vi "Station.vi"() -> ()   [LabVIEW 2016]
uses:
  Station.Data.ctl
  Station.State.ctl
  Sequence/Sequence.State.ctl
  Sequence/Sequence.Test.BreakReason.ctl
  Sequence/Sequence.Test.BreakSource.ctl
  Drivers/FestoCPX/Station/FestoCPX.Station.ProdPresent.ctl
  Drivers/FestoCPX/Station/FestoCPX.Station.EmgState.ctl
  Sequence/Sequence.UserData.ctl
  Sequence/Sequence.MainMode.ctl
  Gui/MainGui.TestOptions.ctl
  Station.Home.Status.Bits.ctl
  Station.Action.ctl
  Drivers/FestoCPX/Station/FestoCPX.Station.TowerLed.Color.ctl
  tools/CitTemplate/citTemplate.errData.ctl
  tools/EventLog/EventLog.EventSource.ctl
  Drivers/FestoCPX/FestoCPX.DO.Signal.ctl
  tools/Translator/Translator.Message.ctl
  Logger/Logger.Variant.Sets.ctl
  Station.Changeover.State.vi
  Station.Plate.Properties.ctl
  Sequence/Sequence.Code.SerialFormat.ctl
  Drivers/V7310/LowLevel/V7310.Job.Sets.ctl
  Drivers/FestoCPX/Station/FestoCPX.Station.ButtonsState.ctl
  Drivers/FestoCPX/Station/FestoCPX.Station.ButtonLed.ctl
  Sequence/Sequence.UserAction.ctl
  Sequence/Sequence.Step.Status.ctl
  Drivers/FestoCPX/Station/FestoCPX.Station.TowerHorn.Fglb.Action.ctl
  Global/ApplicationGlobal.vi
  Station.Global.vi
  tools/Config/Config.Global.vi
  Sequence/Sequence.Global.vi
panel:
  out "action":T1=enum."--- Station ---"
  out "Data":T2
  out "_loop":i32(ring)=4
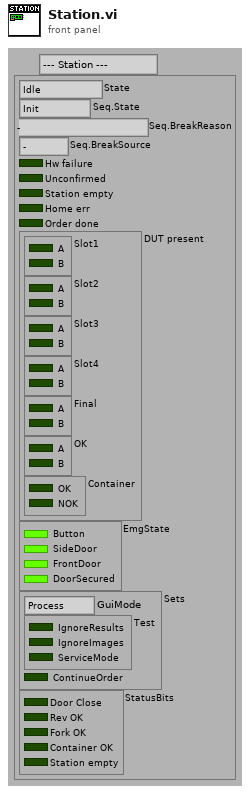
[diagram p1: front panel]
types:
  T1 = typedef "Station.Action.ctl" = enum32{"idle", "constructor", "destructor", "--- Station ---", "Hardware.Init", "Status.Update", "Status.Clear", "Order", "Init", "Ready", "Start", "Run", "Stop", "Error", "Home", "Done", "Seq.Run", "Seq.Done", "Tower.Update", "Mode.Select", "Emg", "Emg.Reset", "Emg.Check", "Home.Check", "Prod.Check", "Butt.Check"}
  T2 = typedef "Station.Data.ctl" = cluster{"State":T3, "Seq.State":T4, "Seq.BreakReason":T5, "Seq.BreakSource":T6, "Hw failure":bool, "Unconfirmed":bool, "Station empty":bool, "Home err":bool, "Order done":bool, "DUT present":T7, "EmgState":T8, "Sets":T9, "StatusBits":T12}
  T3 = typedef "Station.State.ctl" = enum16{"Idle", "Ready", "Run", "Stop", "Error", "Home", "Done", "Emg"}
  T4 = typedef "Sequence.State.ctl" = enum16{"Init", "Idle", "Home", "Work", "Run", "Pause"}
  T5 = typedef "Sequence.Test.BreakReason.ctl" = enum16{"-", "NOK container", "OK container", "Rev empty", "Rev missing", "Rev wrong", "Fork missing", "Fork wrong", "NOK limit", "Unload failure", "Single slot", "Part done", "Err: Prod move work", "Err: Prod move home", "Err: Prod lift work", "Err: Prod lift home", "Err: Prod Arm Work", "Err: Prod Arm NOK", "Err: Prod Arm OK", "Err: Prod NOK suck", "Err: Prod NOK drop", "Err: Prod OK missing", "Err: Prod OK suck", "Err: Prod OK drop"}
  T6 = typedef "Sequence.Test.BreakSource.ctl" = enum16{"-", "A", "B", "A/B"}
  T7 = typedef "FestoCPX.Station.ProdPresent.ctl" = cluster{"Slot1":cluster{"A":bool, "B":bool}, "Slot2":cluster{"A":bool, "B":bool}, "Slot3":cluster{"A":bool, "B":bool}, "Slot4":cluster{"A":bool, "B":bool}, "Final":cluster{"A":bool, "B":bool}, "OK":cluster{"A":bool, "B":bool}, "Container":cluster{"OK":bool, "NOK":bool}}
  T8 = typedef "FestoCPX.Station.EmgState.ctl" = cluster{"Button":bool, "SideDoor":bool, "FrontDoor":bool, "DoorSecured":bool}
  T9 = typedef "Sequence.UserData.ctl" = cluster{"GuiMode":T10, "Test":T11, "ContinueOrder":bool}
  T10 = typedef "Sequence.MainMode.ctl" = enum16{"Process", "Base", "Order", "Manual", "Logs", "Results", "Stats", "DMC Config"}
  T11 = typedef "MainGui.TestOptions.ctl" = cluster{"IgnoreResults":bool, "IgnoreImages":bool, "ServiceMode":bool}
  T12 = typedef "Station.Home.Status.Bits.ctl" = cluster{"Door Close":bool, "Rev OK":bool, "Fork OK":bool, "Container OK":bool, "Station empty":bool}
  T13 = typedef "FestoCPX.Station.TowerLed.Color.ctl" = enum16{"off", "red", "orange", "green", "green/orange"}
  T14 = typedef "citTemplate.errData.ctl" = cluster{"ts":timestamp, "src":T15, "instance":i32, "action":string, "error":errorcluster, "unconfirmed":bool}
  T15 = typedef "EventLog.EventSource.ctl" = enum16{"All", "Gui", "Ref", "File", "Arch", "Seq", "CPX", "DB", "Laser", "Scan.P", "Scan.O"}
  T16 = typedef "FestoCPX.DO.Signal.ctl" = enum16{"Safety Reset", "Air Main Valve", "Door Lock", "Button LED Start", "Button LED Stop", "Button LED Control", "Traffic LED Red", "Traffic LED Orange", "Traffic LED Green", "Horn", "Laser Interlock", "Laser Trigger", "Laser Fume Extractor", "Product Suction Gripper Slot 1 A", "Product Suction Gripper Slot 1 B", "Product Suction Gripper Slot 2 A", "Product Suction Gripper Slot 2 B", "Product Suction Gripper Slot 3 A", "Product Suction Gripper Slot 3 B", "Product Suction Gripper Slot 4 A", "Product Suction Gripper Slot 4 B", "Product Suction Gripper Final A", "Product Suction Gripper Final B", "Lamp", "Q1 Product Move Work", "Q1 Product Move Home", "Q2 Table Turn Work", "Q2 Table Turn Home", "Q3 Product Lift A", "Q3 Product Lift B", "Q4 Product Arm OK", "Q4 Product Arm NOK", "Q5 Product Arm Work", "Q6 Product BlowOut A", "Q6 Product BlowOut B"}
  T17 = typedef "Translator.Message.ctl" = enum16{"-", "Event confirmed", "Log out", "Log in", "Shutdown", "Cancel", "Start", "Begin time", "End time", "Duration", "Service Mode", "Ignore Results", "Serial Format", "On", "Off", "OK", "NOK", "NOK %s", "Home", "Work", "Close", "Open", "In progress...", "Missing", "Empty", "Hardware failure", "Initial", "Default", "Total", "Out of range", "Free disk space is below 1GB - contact technician", "Error %d >> %s", "Error %d >> %s >> %s", "Msg %d >> %s", "Laser msg %d %s", "Laser cmd error %s %d", "Laser cmd failed %s", "Laser cmd warning %s", "Laser disconnected", "Laser status %s", "Laser already started", "Laser job unkonwn %s", "Laser job missing %s", "Laser job select failure %s", "Unable to start laser printing (%s)", "Unable to stop laser printing (%s)", "Laser marking aborted", "Laser marking timeout", "Unable to reset Laser Interlock (%s)", "Unable to trigger Laser. Laser not ready (%s)", "Laser job '%s' coordinates not configured", "Starting %s", "Quitting %s", "Configured", "Initializing", "Quitting", "Loading", "Loaded %d results", "Loaded %d events", "Running", "Stopped", "Summary", "Laser", "Do you want to continue?", "Do you want to delete the configuration?", "The configuration is being used by an order. Unable to delete!", "Press confirm button", "Station is not based. Do you want to exit?", "Station requires changeover. Do you want to run the test?", "Test options are not set as default. Do you want to continue?", "Formatting of WabcoNo is disabled. Do you want to continue?", "Product not detected. Do you want to continue?", "Product scan failed. Do you want to continue?", "Calibration", "Log out?", "System", "All", "IDLE", "Translating...%s", "Not found", "Alarm %s", "Run", "Skip", "Abort", "Repeat", "Please wait...", "Database disconnected", "Database disconnected - changeover disabled!", "Login to database successful", "Login to database failed: %d; %s", "Unable to check the product status of reference %d - database disconnected", "Unable to set the product status of reference %d - database disconnected", "Variant file backup %s", "Read variant (%s)", "Result", "Station armed!", "Station requires changeover!", "Select reference number...", "EMERGENCY BUTTON - press Control button", "EMERGENCY DOOR - press Control button", "Resetting Emergency...", "Unable to reset safety circuit - Emergency Button pressed", "Unable to reset safety circuit - Emergency Side Door open", "Station not based", "Station based", "Station not empty", "Station basing...", "No order", "Press Start to begin new order", "Scanning new order", "Order NOK. Correct or scan again", "Order OK. Press Accept", "Order ready", "Revolver incorrect", "Fork incorrect", "Revolver missing", "Revolver empty", "Container missing", "Offline results", "Offline statistics", "Updating statistics %.1f %%", "DMC Configurator", "Door open", "Close the front door", "Press start button", "Done. Open the front door", "Running...", "Running...%.1f %%", "Pause %s", "Pause %s. NOK container missing", "Pause %s. OK container missing", "Pause %s. Revolver empty", "Pause %s. Revolver missing", "Pause %s. Revolver incorrect", "Pause %s. Fork missing", "Pause %s. Fork incorrect", "Pause %s. Too many failures", "Pause %s. Unloading failure", "Pause %s. One slot is not working", "Pause %s. Part order is done. Empty OK container", "Pause %s. Unable to move product to slot", "Pause %s. Unable to move back product pusher", "Pause %s. Unable to lift product", "Pause %s. Unable to move back product lifter", "Pause %s. Unable to move product arm to Work", "Pause %s. Unable to move product arm to NOK", "Pause %s. Unable to move product arm to OK", "Pause %s. Unable to unsuck the NOK product", "Pause %s. Unable to drop the NOK product", "Pause %s. Product OK missing", "Pause %s. Unable to unsuck the OK product", "Pause %s. Unable to drop the OK product", "Stopping...", "File '%s' is missing", "File '%s' is broken", "File '%s' is running", "Log file started (%s)", "Log file ended (%s)", "Log file stopped (%s)", "Log file ignored (%s)", "Log file exported (%s)", "Log file export failed (%s)", "Wrong serial number in log file", "Wrong reference number in log file", "Test steps are missing", "%s = %.3f", "Process param '%s' not found in DB", "Process param '%s' wrong order", "Process param '%s' value %.3f out of limits (%.3f; %.3f)", "Step%d param '%s' not found in DB", "Step%d param '%s' wrong order", "Step%d param '%s' value %.3f out of limits (%.3f; %.3f)", "Step%d EV '%s' not found in DB", "Step%d EV '%s' wrong order", "\"%s\" not found in DB", "\"%s\" wrong order", "\"%s\" value %.3f out of limits (%.3f; %.3f)", "\"%s\" not found in software", "Process init (%s)", "Process started", "Process restarted", "Process run", "Process done", "Process done - remove OK container", "Process aborted", "Process aborted at work", "Process aborted at home", "Process error", "Process error at home", "Process error at work", "Process close", "Process pause", "Process continue", "Process door open", "Process door close", "Process pause at slot %s due to %s", "Select plate from the order to process", "Do you want to start the process?", "Do you want to continue the process?", "There is unfinished order. Do you want to put the new order?", "Product %s %d OK", "Product %s %d NOK", "Unable to unload the slot %s. Product missing in the slot", "Unable to unload the slot %s. Product already in the arm", "Unable to accept the product as OK. Product missing in slot %s", "Unable to accept the product as OK. Product could not drop into the container at slot %s", "Unable to accept the product as NOK. Product could not drop into the container at slot %s", "Scan failed. Error %s", "Scan failed. Scanner disconnected", "Scan failed. Wrong Wabco number %d, limit (%d,%d)", "Scan failed. Wrong serial number %d, limit (%d,%d)", "Scan failed. Wrong date %d, limit (%d,%d)", "Scan failed. Wrong product wabco number %d (expected %d)", "Scan failed. Wrong product serial number %d (expected > 0)", "Scan OK %s", "Scan failed. Unable to determine table position (%s)", "Scan failed. Timeout", "Tune failed. Scanner disconnected", "Tune failed. Timeout", "%s = %d", "%s = %d->%d", "Unable to set %s = %.2f - Air Pressure Inside off", "Unable to set digital output '%s' = %d", "Unable to activate air pressure inside - timeout", "Unable to activate air pressure inside - aborted", "Unable to switch on Air Main Valve - Air Pressure Inlet off", "Unable to switch on Air Main Valve - Door open", "Unable to switch off Air Main Valve - timeout", "Unable to switch off Air Main Valve - aborted", "Unable to rotate Table - timeout", "Unable to rotate Table - aborted", "Unable to rotate Table - Product Move not in Home position", "Unable to rotate Table - Air Pressure Inside off", "Unable to rotate Table - Product Lift A not in Home position", "Unable to rotate Table - Product Lift B not in Home position", "Unable to rotate Table - unlock before movement timeout", "Unable to rotate Table - lock after movement timeout", "Unable to move Table Lock to %s position - timeout", "Unable to move Table Lock to %s position - aborted", "Unable to move Table Lock to %s position - Air Pressure Inside off", "Unable to move Table Lock to %s position - Table not in position", "Unable to move Product Lift A to %s position - timeout", "Unable to move Product Lift B to %s position - timeout", "Unable to move Product Lift A to %s position - aborted", "Unable to move Product Lift B to %s position - aborted", "Unable to move Product Lift A to %s position - Air Pressure Inside off", "Unable to move Product Lift B to %s position - Air Pressure Inside off", "Unable to move Product Lift A to %s position - Table not locked", "Unable to move Product Lift B to %s position - Table not locked", "Unable to move Product Lift A to %s position - Product Arm not in Work position", "Unable to move Product Lift B to %s position - Product Arm not in Work position", "Unable to set Product Suction Gripper %s to %s - timeout", "Unable to set Product Suction Gripper %s to %s - aborted", "Unable to set Product Suction Gripper %s to %s - Air Pressure Inside off", "Unable to set Product Suction Gripper %s to %s - Table slot unkown", "Unable to move Product Arm to %s position - timeout", "Unable to move Product Arm to %s position - aborted", "Unable to move Product Arm to %s position - Air Pressure Inside off", "Unable to move Product Arm to %s position - Product Lift A not in Home position", "Unable to move Product Arm to %s position - Product Lift B not in Home position", "Unable to move Product to %s position - timeout", "Unable to move Product to %s position - aborted", "Unable to move Product to %s position - Air Pressure Inside off", "Unable to move Product to %s position - Table not in position"}
  T18 = typedef "Logger.Variant.Sets.ctl" = cluster{"State":T19, "ImgPath":path, "WabcoPlate":string, "WabcoProduct":string, "ClientProduct":string, "ClientPlate":string, "TotalQuantity":u16, "OrderQuantity":u16, "Serial":i32, "Wabco":T20, "Client":T20}
  T19 = typedef "Station.Changeover.State.vi" = enum16{"Init", "Scaning", "NOK", "Wait for ack", "Ready"}
  T20 = typedef "Station.Plate.Properties.ctl" = cluster{"LaserJob":string, "AdditionalTxt":string, "FactoryCode":string, "RevID":u8, "ForkID":u8, "FailuresLimit":u16, "GlobalCnt":i32, "Bank":u8, "SerialFormat":T21, "CoordA":T22, "CoordB":T22, "DMCconfig":i32}
  T21 = typedef "Sequence.Code.SerialFormat.ctl" = enum8{"", "6 dig", "7 dig"}
  T22 = typedef "V7310.Job.Sets.ctl" = cluster{"X":dbl, "Y":dbl, "Angle":dbl}
  T23 = typedef "FestoCPX.Station.ButtonsState.ctl" = cluster{"Start":bool, "Stop":bool, "Control":bool}
  T24 = typedef "Sequence.UserAction.ctl" = enum16{"-", "Stop", "Pause", "Continue", "Next"}
  T25 = typedef "FestoCPX.Station.ButtonLed.ctl" = enum16{"Start", "Stop", "Control"}
  T26 = cluster{"State":T4, "PauseReason":T5, "BreakSource":T6}
  T27 = typedef "Sequence.Step.Status.ctl" = enum16{"-", "Pending", "Running", "Skipped", "Passed", "Failed", "Done", "Error", "Aborted", "Stopped"}
  T28 = cluster{"State":T4, "Status":T27, "order done":bool}
  T29 = typedef "FestoCPX.Station.TowerHorn.Fglb.Action.ctl" = enum16{"init", "set", "get"}
  T30 = typedef "citTemplate.notifierHandle.ctl" = refnum<notifier>
  T31 = cluster{"Arguments":variant[], "msg":T17, "BgColor":u32, u32, "Blink":bool}
  T32 = typedef "Sequence.Data.ctl" = cluster{"BeginTS":timestamp, "EndTS":timestamp, "State":T4, "Status.Work":T27, "Status.Process":T27, "Status.Home":T27, "Status.Wabco":T27, "Status.Client":T27, "BreakReason":T5, "BreakSource":T6, "DoorLock":bool, "Status.Prod":T33[], "UserAction":T37, "UserData":T9, "Error":errorcluster, "Code":T38, "Rotations":i32, "ProdIdx":i32, "ProdDone":T33[], "PrintedSerials-Wabco":i32[], "PrintedSerials-Client":i32[], "Counters-Wabco":T40, "Counters-Client":T40}
  T33 = typedef "Sequence.Test.Status.ctl" = cluster{"Slot":T34, "A":T36, "B":T36}
  T34 = typedef "Sequence.Slot.StatusData.ctl" = cluster{"ID":i32, "Unload":T35, "TS":timestamp, "duration":u32}
  T35 = typedef "Sequence.Test.Unload.Status.ctl" = enum16{"init", "check NOK", "check OK", "wait on NOK", "wait on OK", "wait on Unload", "done"}
  T36 = typedef "Sequence.Prod.StatusData.ctl" = cluster{"status":T27, "pause":T5, "present":bool, "printed":bool, "scanned":bool, "tuned":bool, "removed":bool, "LaserVariables":string[], "ScanerReadOut":string, "path":path, "corners":cluster{"X":i32, "Y":i32}[], "verification":u8}
  T37 = typedef "Sequence.UserActions.ctl" = cluster{"Stop":bool, "Pause":bool, "Next":bool}
  T38 = typedef "Sequence.Code.Sets.ctl" = cluster{"Ready":bool, "DoubleOrder":bool, "OrderDone":bool, "AllowSingleSlot":bool, "CheckDM":bool, "ThresholdA":u8, "ThresholdB":u8, "Plate":T39, "ImgPath":path, "Variant":T18}
  T39 = typedef "Sequence.PlateType.ctl" = enum16{"Wabco", "Client"}
  T40 = typedef "Sequence.Counters.ctl" = cluster{"Expected":u16, "Done":u16, "OK":u16, "NOK":u16, "NOKlimit":u16, "Part":u16, "PartOK":u16}
  T41 = typedef "Station.Buttons.ctl" = cluster{"Start":bool, "Stop":bool, "Control":bool}
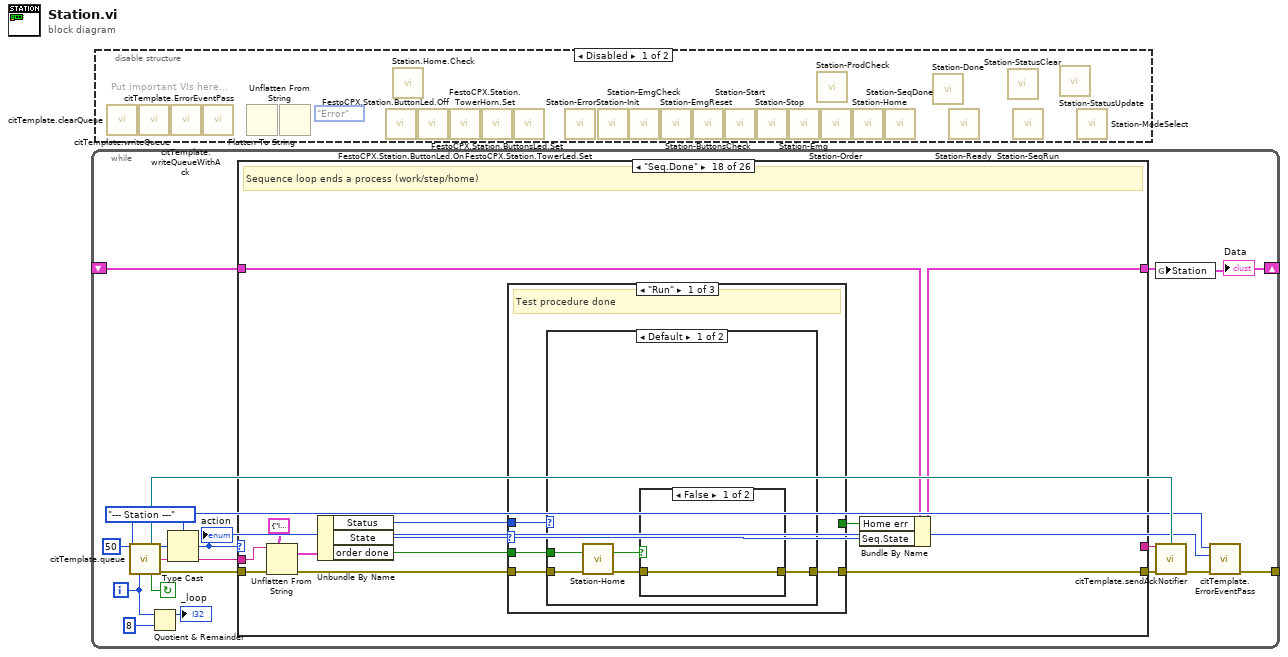
[diagram p0: block diagram]
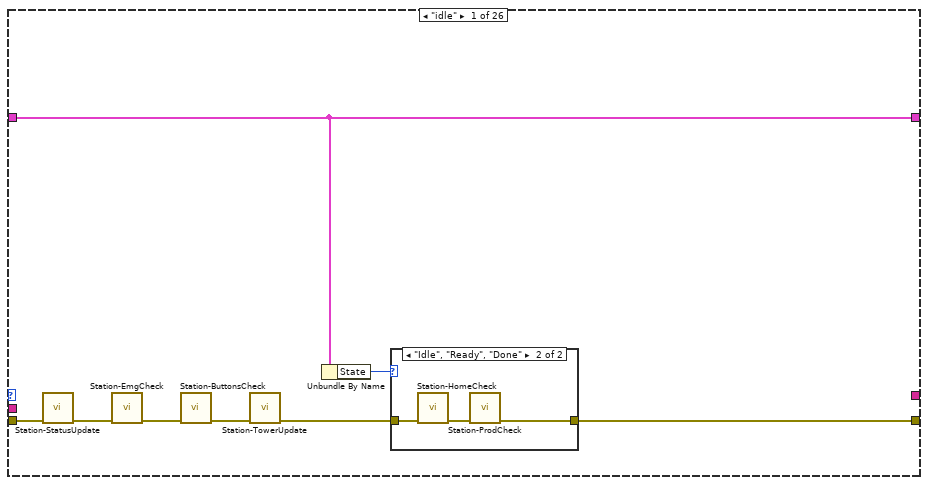
[diagram p3: hidden frame]
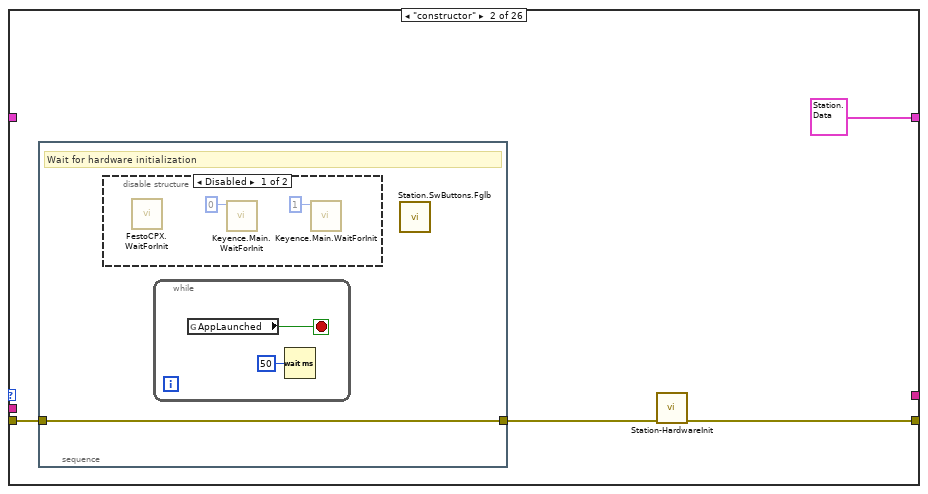
[diagram p5: hidden frame]
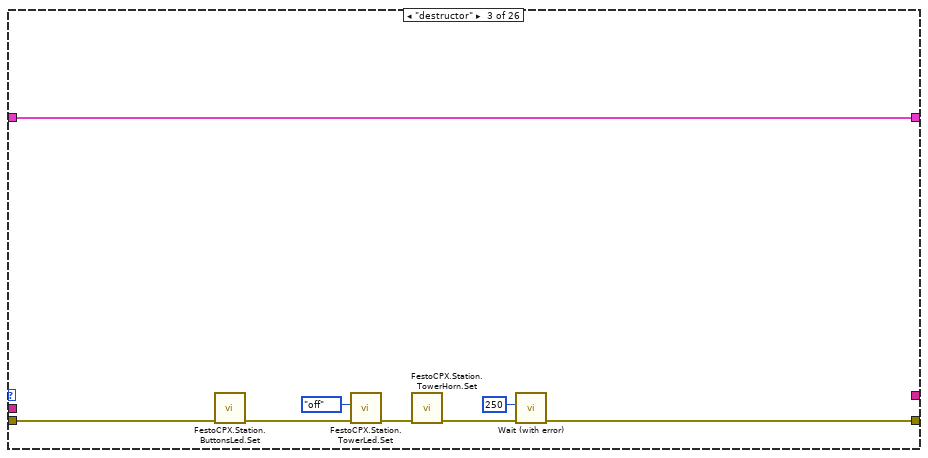
[diagram p7: hidden frame]
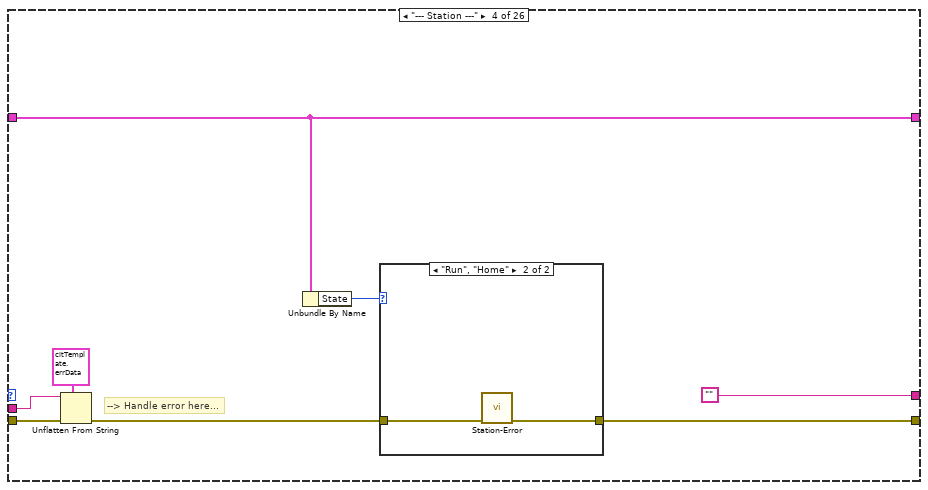
[diagram p8: hidden frame]
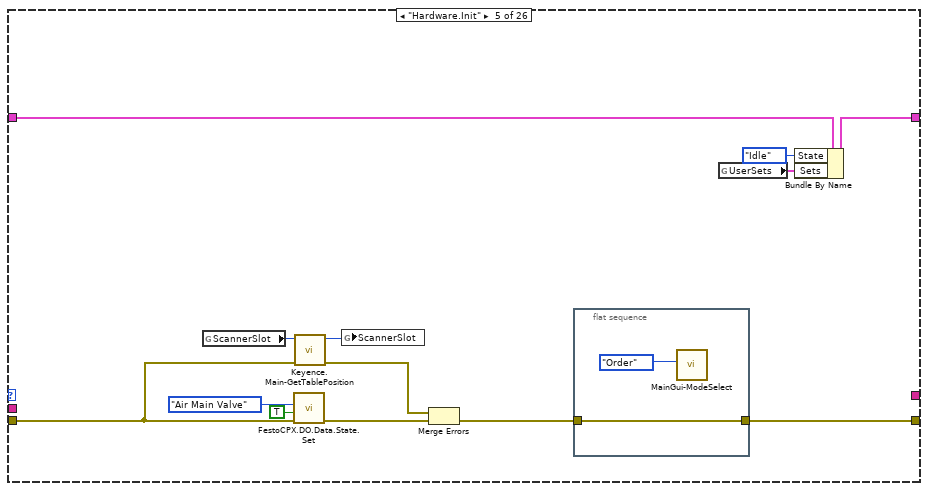
[diagram p10: hidden frame]
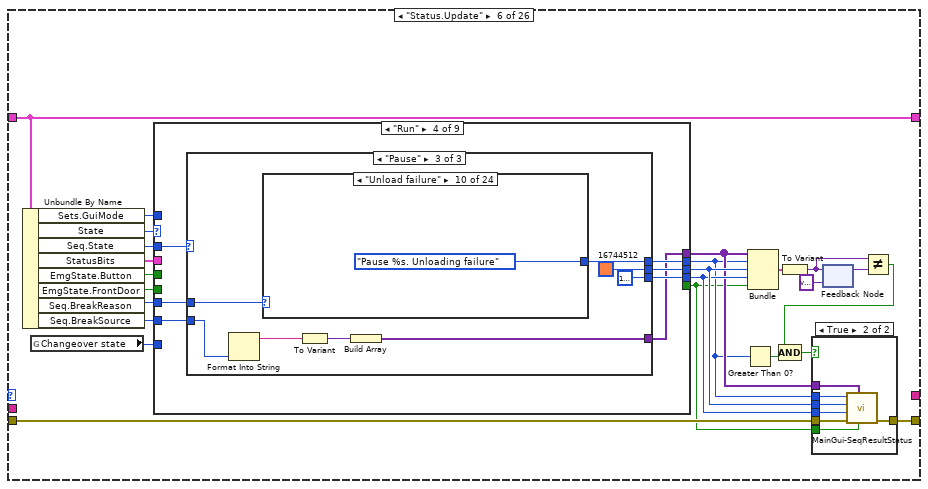
[diagram p11: hidden frame]
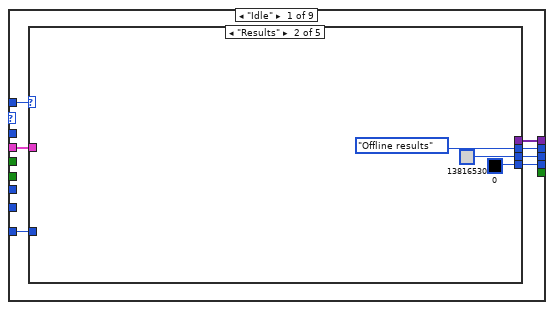
[diagram p13: hidden frame]
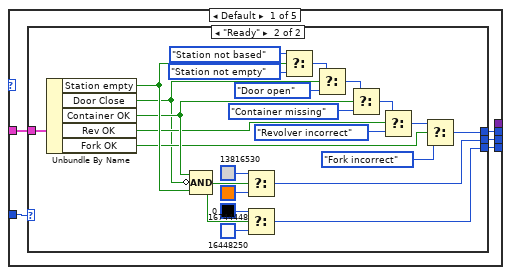
[diagram p14: hidden frame]
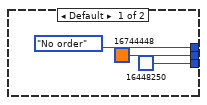
[diagram p15: hidden frame]
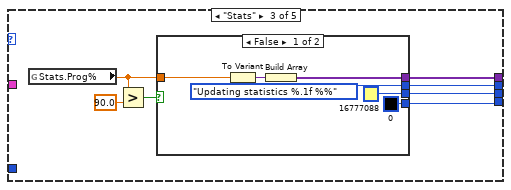
[diagram p16: hidden frame]
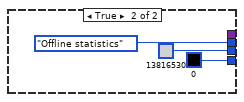
[diagram p17: hidden frame]
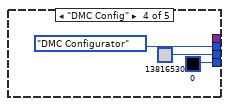
[diagram p18: hidden frame]
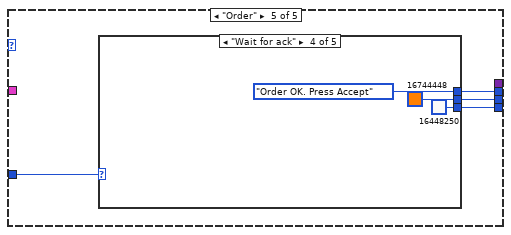
[diagram p19: hidden frame]
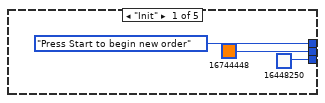
[diagram p20: hidden frame]
diagram:
  n1 = while {
    tunnel: [w5] -> _
    shift-right: [w2] -> _
    shift-left: _ -> [w3]
    i -> [w7]
    stop <- w13 continue-if-true
    w10 = Station.Action."--- Station ---" ("Action")
    n2 = call "citTemplate.queue.vi"("ms timeout (250 ms)"=50, "event enum"=w10, "iteration (-1)"=w7) -> ("notifierHandle out"=w12:T30, "event out"=w16:u32, "(flatten) data out"=w15:string, "continue"=w13:bool, "error out"=w14:errorcluster)  [unwired: 2 in, 6 out]
    n3 = Quotient & Remainder(x=w7, y=8) -> (x-y*floor(x/y)=→"_loop":i32)  [unwired: 1 out]
    n4 = Type Cast(type=w10, x=w16) -> (*(type *) &x=w6:T1)
    "action" <- w6
    n5 = case shown="\"Seq.Done\"" w6 {
      tunnel: w15 -> [_ _ _ w52 _ _ _ w304 _ _ _ _ _ _ _ _ w443 w466 _ w525 _ _ _ _ _ _]
      tunnel: w14 -> [w24 w32 w38 w51 w65 w89 w289 w311 w335 w345 w365 w388 w399 w405 w417 w430 w444 w467 w502 w526 w549 w568 w587 w613 w643 w663]
      tunnel: [_ _ _ "" _ _ _ _ _ _ _ _ _ _ _ _ _ _ _ _ _ _ _ _ _ _] -> w11
      tunnel: [w22 T2 {"State"=enum."Idle", "Seq.State"=enum."Init", "Seq.BreakReason"=enum."-", "Seq.BreakSource"=enum."-", "Hw failure"=FALSE, "Unconfirmed"=FALSE, "Station empty"=FALSE, "Home err"=FALSE, "Order done"=FALSE, "DUT present"={"Slot1"={"A"=FALSE, "B"=FALSE}, "Slot2"={"A"=FALSE, "B"=FALSE}, "Slot3"={"A"=FALSE, "B"=FALSE}, "Slot4"={"A"=FALSE, "B"=FALSE}, "Final"={"A"=FALSE, "B"=FALSE}, "OK"={"A"=FALSE, "B"=FALSE}, "Container"={"OK"=FALSE, "NOK"=FALSE}}, "EmgState"={"Button"=FALSE, "SideDoor"=FALSE, "FrontDoor"=FALSE, "DoorSecured"=FALSE}, "Sets"={"GuiMode"=enum."Process", "Test"={"IgnoreResults"=FALSE, "IgnoreImages"=FALSE, "ServiceMode"=FALSE}, "ContinueOrder"=FALSE}, "StatusBits"={"Door Close"=FALSE, "Rev OK"=FALSE, "Fork OK"=FALSE, "Container OK"=FALSE, "Station empty"=FALSE}} ("Data") w42 w49 w59 w95 w294 w306 w339 w352 w360 w390 w400 w410 w421 w433 w442 w461 w505 w518 w554 w569 w582 w611 w641 w649] -> w2
      tunnel: w3 -> [w22 _ w42 w49 w60 w95 w291 w306 w337 w350 w362 w387 w398 w404 w420 w431 w441 w457 w505 w523 w548 w570 w583 w612 w640 w649]
      tunnel: [w17 w30 w44 w47 w57 w90 w292 w309 w334 w344 w364 w384 w391 w403 w419 w424 w436 w463 w494 w520 w547 w566 w585 w610 w642 w653] -> w1
      frame "idle" {
        n6 = call "Station-StatusUpdate.vi"("error in (no error)"=w24) -> ("error out"=w23:errorcluster)  [unwired: 10 in]
        n7 = call "Station-EmgCheck.vi"("error in (no error)"=w23) -> ("error out"=w20:errorcluster)  [unwired: 10 in]
        n8 = call "Station-ButtonsCheck.vi"("error in (no error)"=w20) -> ("error out"=w19:errorcluster)  [unwired: 10 in]
        n9 = call "Station-TowerUpdate.vi"("error in (no error)"=w19) -> ("error out"=w18:errorcluster)  [unwired: 10 in]
        n10 = Unbundle By Name(w22) -> ("State"=w21:T3)
        n11 = case shown="\"Idle\", \"Ready\", \"Done\"" w21 {
          tunnel: w18 -> [w25 w28]
          tunnel: [w25 w26] -> w17
          frame Default {
          }
          frame "Idle", "Ready", "Done" {
            n12 = call "Station-HomeCheck.vi"("error in (no error)"=w28) -> ("error out"=w27:errorcluster)  [unwired: 10 in]
            n13 = call "Station-ProdCheck.vi"("error in (no error)"=w27) -> ("error out"=w26:errorcluster)  [unwired: 10 in]
          }
        }
      }
      frame "constructor" {
        n14 = stacked-sequence {
          tunnel: w32 -> [w33]
          tunnel: [w33] -> w31
          frame #0 {
            # "Wait for hardware initialization"
            n15 = disable-structure shown="Disabled" {
              frame Disabled {
                n16 = call "FestoCPX.WaitForInit.vi"() -> ()  [unwired: 12 in]
                n17 = call "Keyence.Main.WaitForInit.vi"("idx"=0) -> ()  [unwired: 11 in]
                n18 = call "Keyence.Main.WaitForInit.vi"("idx"=1) -> ()  [unwired: 11 in]
              }
              frame Enabled {
              }
            }
            n19 = while {
              stop <- w35 stop-if-true
              n20 = global read "ApplicationGlobal.vi" "AppLaunched"() -> (w35:bool)
              n21 = Wait (ms)(milliseconds to wait=u32 50) -> ()  [unwired: 1 out]
            }
            n22 = call "Station.SwButtons.Fglb.vi"() -> ()  [unwired: 2 in, 1 out]
          }
        }
        n23 = call "Station-HardwareInit.vi"("error in (no error)"=w31) -> ("error out"=w30:errorcluster)  [unwired: 10 in]
      }
      frame "destructor" {
        n24 = call "FestoCPX.Station.ButtonsLed.Set.vi"("error in"=w38) -> ("error out"=w39:errorcluster)  [unwired: 10 in]
        n25 = call "FestoCPX.Station.TowerLed.Set.vi"("error in"=w39, "Color (off)"=FestoCPX.Station.TowerLed.Color."off") -> ("error out"=w40:errorcluster)  [unwired: 9 in]
        n26 = call "FestoCPX.Station.TowerHorn.Set.vi"("error in"=w40) -> ("error out"=w45:errorcluster)  [unwired: 10 in]
        n27 = call "Wait (with error).vi"("error in (no error)"=w45, "milliseconds to wait"=u32 250) -> ("error out"=w44:errorcluster)  [unwired: 8 in, 1 out]
      }
      frame "--- Station ---" {
        # "--> Handle error here..."
        n28 = Unflatten From String(type=T14 {"ts"=timestamp(0 s since 1904-01-01), "src"=enum."All", "instance"=0, "action"="", "error"={"status"=FALSE, "code"=0, "source"=""}, "unconfirmed"=FALSE} ("ErrData"), binary string=w52, error in (no error)=w51) -> (error out=w46:errorcluster)  [unwired: 4 out]
        n29 = Unbundle By Name(w49) -> ("State"=w48:T3)
        n30 = case shown="\"Run\", \"Home\"" w48 {
          tunnel: w46 -> [w54 w56]
          tunnel: [w54 w55] -> w47
          frame Default {
          }
          frame "Run", "Home" {
            n31 = call "Station-Error.vi"("error in (no error)"=w56) -> ("error out"=w55:errorcluster)  [unwired: 10 in]
          }
        }
      }
      frame "Hardware.Init" {
        n32 = global read "Station.Global.vi" "ScannerSlot"() -> (w67:i32)
        n33 = call "FestoCPX.DO.Data.State.Set.vi"("error in (no error)"=w65, "State"=TRUE, "CPX.DO"=FestoCPX.DO.Signal."Air Main Valve") -> ("error out"=w64:errorcluster)  [unwired: 8 in]
        n34 = call "Keyence.Main-GetTablePosition.vi"("error in (no error)"=w65, "ScannerSlot in"=w67) -> ("error out"=w63:errorcluster, "ScannerSlot out"=w66:i32)  [unwired: 7 in, 1 out]
        n35 = global write "Station.Global.vi" "ScannerSlot"(w66) -> ()
        n36 = Merge Errors(w63, w64) -> (w58:errorcluster)
        n37 = flat-sequence {
          tunnel: w58 -> [w70]
          tunnel: [w70] -> w57
          frame #0 {
            n38 = call "MainGui-ModeSelect.vi"("Mode"=Sequence.MainMode."Order" ("f")) -> ()  [unwired: 10 in, 1 out]
          }
        }
        n39 = global read "Config.Global.vi" "UserSets"() -> (w62:T9)
        n40 = Bundle By Name(cluster=w60, "State"=Station.State."Idle", "Sets"=w62) -> (w59:T2)
      }
      frame "Status.Update" {
        n41 = Unbundle By Name(w95) -> ("Sets.GuiMode"=w76:T10, "State"=w94:T3, "Seq.State"=w77:T4, "StatusBits"=w78:T12, "EmgState.Button"=w81:bool, "EmgState.FrontDoor"=w74:bool, "Seq.BreakReason"=w75:T5, "Seq.BreakSource"=w72:T6)
        n42 = global read "Station.Global.vi" "Changeover state"() -> (w73:T19)
        n43 = case shown="\"Run\"" w94 {
          tunnel: [w110 w189 Translator.Message."Done. Open the front door" ("msg") w235 Translator.Message."Stopping..." ("msg") _ Translator.Message."Station basing..." ("msg") w281 _] -> w85
          tunnel: [w109 w188 u32 16744448 w234 u32 16860 _ u32 16860 u32 16711680 _] -> w88
          tunnel: [w108 w187 u32 16448250 w233 u32 16448250 _ u32 16448250 u32 16777225 _] -> w87
          tunnel: [w104 w184 _ w229 _ _ _ _ variant[] [] ("Arguments")] -> w86
          tunnel: [_ _ _ _ _ _ _ TRUE ("Blink") _] -> w79
          tunnel: w81 -> [_ _ _ _ _ _ _ w282 _]
          tunnel: w78 -> [w107 w186 _ _ _ _ _ _ _]
          tunnel: w77 -> [_ _ _ w232 _ _ _ _ _]
          tunnel: w76 -> [w106 w185 _ _ _ _ _ _ _]
          tunnel: w75 -> [_ _ _ w231 _ _ _ _ _]
          tunnel: w74 -> [_ _ _ _ _ _ _ _ _]
          tunnel: w73 -> [w105 _ _ _ _ _ _ _ _]
          tunnel: w72 -> [_ _ _ w230 _ _ _ _ _]
          frame "Idle" {
            n44 = case shown="\"Results\"" w106 {
              tunnel: [w115 Translator.Message."Offline results" ("msg") w150 Translator.Message."DMC Configurator" ("msg") w168] -> w110
              tunnel: [w114 u32 13816530 w149 u32 13816530 w167] -> w109
              tunnel: [w113 u32 0 w148 u32 0 w166] -> w108
              tunnel: w107 -> [w112 _ _ _ _]
              tunnel: w105 -> [w111 _ _ _ w165]
              tunnel: [_ _ w147 _ _] -> w104
              frame Default {
                n45 = case shown="\"Ready\"" w111 {
                  tunnel: [Translator.Message."No order" ("msg") w120] -> w115
                  tunnel: [u32 16744448 w130] -> w114
                  tunnel: [u32 16448250 w129] -> w113
                  tunnel: w112 -> [_ w128]
                  frame Default {
                  }
                  frame "Ready" {
                    n46 = Unbundle By Name(w128) -> ("Station empty"=w134:bool, "Door Close"=w119:bool, "Container OK"=w127:bool, "Rev OK"=w126:bool, "Fork OK"=w122:bool)
                    n47 = Compound Arithmetic op=AND(w127, invert w119, w134) -> (w131:bool)
                    n48 = Select(t=u32 13816530, s=w131, f=u32 16744448) -> (s? t:f=w130:u32)
                    n49 = Select(t=u32 0, s=w131, f=u32 16448250) -> (s? t:f=w129:u32)
                    n50 = Select(t=Translator.Message."Station not based" ("msg"), s=w134, f=Translator.Message."Station not empty" ("msg")) -> (s? t:f=w139:T17)
                    n51 = Select(t=w139, s=w119, f=Translator.Message."Door open" ("msg")) -> (s? t:f=w140:T17)
                    n52 = Select(t=w140, s=w127, f=Translator.Message."Container missing" ("msg")) -> (s? t:f=w124:T17)
                    n53 = Select(t=w124, s=w126, f=Translator.Message."Revolver incorrect" ("msg")) -> (s? t:f=w123:T17)
                    n54 = Select(t=w123, s=w122, f=Translator.Message."Fork incorrect" ("msg")) -> (s? t:f=w120:T17)
                  }
                }
              }
              frame "Results" {
              }
              frame "Stats" {
                n55 = global read "ApplicationGlobal.vi" "Stats.Prog%"() -> (w146:dbl)
                n56 = Greater?(x=w146, y=90.0) -> (0:w151:bool)
                n57 = case shown="False" w151 {
                  tunnel: [Translator.Message."Updating statistics %.1f %%" ("msg") Translator.Message."Offline statistics" ("msg")] -> w150
                  tunnel: [u32 16777088 u32 13816530] -> w149
                  tunnel: [u32 0 u32 0] -> w148
                  tunnel: [w156 _] -> w147
                  tunnel: w146 -> [w155 _]
                  frame False {
                    n58 = To Variant(anything=w155) -> (Variant=w157:variant)
                    n59 = Build Array(w157) -> (w156:variant[])
                  }
                  frame True {
                  }
                }
              }
              frame "DMC Config" {
              }
              frame "Order" {
                n60 = case shown="\"Wait for ack\"" w165 {
                  tunnel: [Translator.Message."Press Start to begin new order" ("msg") Translator.Message."Order NOK. Correct or scan again" ("msg") Translator.Message."Scanning new order" ("msg") Translator.Message."Order OK. Press Accept" ("msg") Translator.Message."Order ready" ("msg")] -> w168
                  tunnel: [u32 16744448 u32 16744448 u32 16744448 u32 16744448 u32 13816530] -> w167
                  tunnel: [u32 16448250 u32 16448250 u32 16448250 u32 16448250 u32 0] -> w166
                  frame "Init" {
                  }
                  frame "NOK" {
                  }
                  frame "Scaning" {
                  }
                  frame "Wait for ack" {
                  }
                  frame "Ready" {
                  }
                }
              }
            }
          }
          frame "Ready" {
            n61 = case shown="\"Results\"" w185 {
              tunnel: [_ w192 w210 Translator.Message."Station based" ("msg") Translator.Message."Offline results" ("msg") Translator.Message."Press Start to begin new order" ("msg")] -> w189
              tunnel: [_ w190 w209 u32 13816530 u32 13816530 u32 13816530] -> w188
              tunnel: [_ w193 w208 u32 0 u32 0 u32 0] -> w187
              tunnel: w186 -> [_ _ w207 _ _ _]
              tunnel: [_ w191 _ _ _ _] -> w184
              frame Default {
              }
              frame "Stats" {
                n62 = global read "ApplicationGlobal.vi" "Stats.Prog%"() -> (w194:dbl)
                n63 = Greater?(x=w194, y=90.0) -> (0:w195:bool)
                n64 = case shown="False" w195 {
                  tunnel: [Translator.Message."Updating statistics %.1f %%" ("msg") Translator.Message."Offline statistics" ("msg")] -> w192
                  tunnel: [u32 16777088 u32 13816530] -> w190
                  tunnel: [u32 0 u32 0] -> w193
                  tunnel: [w200 _] -> w191
                  tunnel: w194 -> [w199 _]
                  frame False {
                    n65 = To Variant(anything=w199) -> (Variant=w201:variant)
                    n66 = Build Array(w201) -> (w200:variant[])
                  }
                  frame True {
                  }
                }
              }
              frame "Process" {
                n67 = Unbundle By Name(w207) -> ("Door Close"=w206:bool)
                n68 = case shown="False" w206 {
                  tunnel: [Translator.Message."Close the front door" ("msg") Translator.Message."Press start button" ("msg")] -> w210
                  tunnel: [u32 13816530 u32 13816530 ("BgColor")] -> w209
                  tunnel: [u32 0 u32 0] -> w208
                  frame False {
                  }
                  frame True {
                  }
                }
              }
              frame "Base" {
              }
              frame "Results" {
              }
              frame "Order" {
              }
            }
          }
          frame "Done" {
          }
          frame "Run" {
            n69 = case shown="\"Pause\"" w232 {
              tunnel: [Translator.Message."Running..." ("msg") Translator.Message."Running..." ("msg") w247] -> w235
              tunnel: [u32 16860 u32 16860 u32 16744512] -> w234
              tunnel: [u32 16777225 u32 16777225 u32 16777225] -> w233
              tunnel: w231 -> [_ _ w246]
              tunnel: w230 -> [_ _ w245]
              tunnel: [_ _ w242] -> w229
              frame Default {
              }
              frame "Run" {
              }
              frame "Pause" {
                n70 = Format Into String(w245) -> (resulting string=w244:string)  [unwired: 3 in, 1 out]
                n71 = case shown="\"Unload failure\"" w246 {
                  tunnel: [Translator.Message."Pause %s" ("msg") Translator.Message."Pause %s. NOK container missing" ("msg") Translator.Message."Pause %s. OK container missing" ("msg") Translator.Message."Pause %s. Revolver empty" ("msg") Translator.Message."Pause %s. Revolver missing" ("msg") Translator.Message."Pause %s. Revolver incorrect" ("msg") Translator.Message."Pause %s. Fork missing" ("msg") Translator.Message."Pause %s. Fork incorrect" ("msg") Translator.Message."Pause %s. Too many failures" ("msg") Translator.Message."Pause %s. Unloading failure" ("msg") Translator.Message."Pause %s. One slot is not working" ("msg") Translator.Message."Pause %s. Part order is done. Empty OK container" ("msg") Translator.Message."Pause %s. Unable to move product to slot" ("msg") Translator.Message."Pause %s. Unable to move back product pusher" ("msg") Translator.Message."Pause %s. Unable to lift product" ("msg") Translator.Message."Pause %s. Unable to move back product lifter" ("msg") Translator.Message."Pause %s. Unable to move product arm to Work" ("msg") Translator.Message."Pause %s. Unable to move product arm to NOK" ("msg") Translator.Message."Pause %s. Unable to move product arm to OK" ("msg") Translator.Message."Pause %s. Unable to unsuck the NOK product" ("msg") Translator.Message."Pause %s. Unable to drop the NOK product" ("msg") Translator.Message."Pause %s. Product OK missing" ("msg") Translator.Message."Pause %s. Unable to unsuck the OK product" ("msg") Translator.Message."Pause %s. Unable to drop the OK product" ("msg")] -> w247
                  frame "-" {
                  }
                  frame "NOK container" {
                  }
                  frame "OK container" {
                  }
                  frame "Rev empty" {
                  }
                  frame "Rev missing" {
                  }
                  frame "Rev wrong" {
                  }
                  frame "Fork missing" {
                  }
                  frame "Fork wrong" {
                  }
                  frame "NOK limit" {
                  }
                  frame "Unload failure" {
                  }
                  frame "Single slot" {
                  }
                  frame "Part done" {
                  }
                  frame "Err: Prod move work" {
                  }
                  frame "Err: Prod move home" {
                  }
                  frame "Err: Prod lift work" {
                  }
                  frame "Err: Prod lift home" {
                  }
                  frame "Err: Prod Arm Work" {
                  }
                  frame "Err: Prod Arm NOK" {
                  }
                  frame "Err: Prod Arm OK" {
                  }
                  frame "Err: Prod NOK suck" {
                  }
                  frame "Err: Prod NOK drop" {
                  }
                  frame "Err: Prod OK missing" {
                  }
                  frame "Err: Prod OK suck" {
                  }
                  frame "Err: Prod OK drop" {
                  }
                }
                n72 = To Variant(anything=w244) -> (Variant=w243:variant)
                n73 = Build Array(w243) -> (w242:variant[])
              }
            }
          }
          frame "Stop" {
          }
          frame "Error" {
          }
          frame "Home" {
          }
          frame "Emg" {
            n74 = Select(t=Translator.Message."EMERGENCY BUTTON - press Control button" ("msg"), s=w282, f=Translator.Message."EMERGENCY DOOR - press Control button" ("msg")) -> (s? t:f=w281:T17)
          }
          frame Default {
          }
        }
        n75 = Greater Than 0?(x=w85) -> (x > 0?=w84:bool)
        n76 = Bundle("Arguments"=w86, "msg"=w85, "BgColor"=w88, w87, "Blink"=w79) -> (w93:T31)  [unwired: 1 in]
        n77 = To Variant(anything=w93) -> (Variant=w91:variant)
        n78 = feedback-in #1(w91) -> ()
        n79 = feedback #1(variant ("Variant")) -> (w92:variant)
        n80 = Not Equal?(x=w91, y=w92) -> (x != y?=w83:bool)
        n81 = Compound Arithmetic op=AND(w83, w84) -> (w82:bool)
        n82 = case shown="True" w82 {
          tunnel: [w96 w103] -> w90
          tunnel: w89 -> [w96 w102]
          tunnel: w88 -> [_ w101]
          tunnel: w87 -> [_ w100]
          tunnel: w85 -> [_ w99]
          tunnel: w86 -> [_ w98]
          tunnel: w79 -> [_ w97]
          frame False {
          }
          frame True {
            n83 = call "MainGui-SeqResultStatus.vi"("Blink"=w97, "Arguments"=w98, "error in (no error)"=w102, "TxtColor"=w100, "BgColor"=w101, "Msg"=w99) -> ("error out"=w103:errorcluster)  [unwired: 5 in]
          }
        }
      }
      frame "Status.Clear" {
        n84 = call "ErrorHandling.Fglb.Confirm.vi"("error in (no error)"=w289) -> ("error out"=w288:errorcluster)  [unwired: 10 in]
        n85 = call "FestoCPX.Station.TowerHorn.Set.vi"("error in"=w288) -> ("error out"=w296:errorcluster)  [unwired: 10 in]
        n86 = call "Sequence-StatusClear.vi"("error in (no error)"=w296) -> ("error out"=w293:errorcluster)  [unwired: 10 in]
        n87 = Unbundle By Name(w291) -> ("Home err"=w290:bool)
        n88 = case shown="True" w290 {
          tunnel: w293 -> [w298 w300]
          tunnel: [w297 w299] -> w292
          frame False {
            n89 = call "Station-Home.vi"("error in (no error)"=w298) -> ("error out"=w297:errorcluster)  [unwired: 10 in]
          }
          frame True {
            n90 = call "Station-Done.vi"("error in (no error)"=w300) -> ("error out"=w299:errorcluster)  [unwired: 10 in]
          }
        }
        n91 = Bundle By Name(cluster=w291, "Unconfirmed"=FALSE) -> (w294:T2)
      }
      frame "Order" {
        # "Select reference"
        n92 = Unflatten From String(type=T18 {"State"=enum."Init", "ImgPath"=path "", "WabcoPlate"="", "WabcoProduct"="", "ClientProduct"="", "ClientPlate"="", "TotalQuantity"=0, "OrderQuantity"=0, "Serial"=0, "Wabco"={"LaserJob"="", "AdditionalTxt"="037", "FactoryCode"="", "RevID"=0, "ForkID"=0, "FailuresLimit"=0, "GlobalCnt"=0, "Bank"=0, "SerialFormat"=enum."6 dig", "CoordA"={"X"=0.0, "Y"=0.0, "Angle"=0.0}, "CoordB"={"X"=0.0, "Y"=0.0, "Angle"=0.0}, "DMCconfig"=0}, "Client"={"LaserJob"="", "AdditionalTxt"="", "FactoryCode"="037", "RevID"=0, "ForkID"=0, "FailuresLimit"=0, "GlobalCnt"=0, "Bank"=0, "SerialFormat"=enum."6 dig", "CoordA"={"X"=0.0, "Y"=0.0, "Angle"=0.0}, "CoordB"={"X"=0.0, "Y"=0.0, "Angle"=0.0}, "DMCconfig"=0}} ("VariantSets"), binary string=w304, error in (no error)=w311) -> (value=w302:T18, error out=w305:errorcluster)  [unwired: 2 in, 1 out]
        n93 = global read "Sequence.Global.vi" "SeqData"() -> (w308:T32)
        n94 = call "Station-Init.vi"("error in (no error)"=w305) -> ("error out"=w310:errorcluster)  [unwired: 10 in]
        n95 = Unbundle By Name(w308) -> ("Status.Process"=w307:T27)
        n96 = Unbundle By Name(w302) -> ("State"=w301:T19)
        n97 = case shown="\"Ready\"" w301 {
          tunnel: [w312 w318] -> w309
          tunnel: w310 -> [w313 w320]
          tunnel: w302 -> [_ w319]
          tunnel: w307 -> [_ w317]
          frame Default {
            n98 = call "MainGui-ModeSelect.vi"("error in (no error)"=w313, "Mode"=Sequence.MainMode."Order" ("f")) -> ("error out"=w312:errorcluster)  [unwired: 9 in]
          }
          frame "Ready" {
            n99 = case shown="\"Pending\", \"Running\", \"Error\"..\"Stopped\"" w317 {
              tunnel: [TRUE ("ok") w323] -> w316
              tunnel: Translator.Message."There is unfinished order. Do you want to put the new order?" ("_Msg") -> [_ w322]
              frame Default {
              }
              frame "Pending", "Running", "Error".."Stopped" {
                n100 = call "InfoGui.vi"("_Msg"=w322) -> ("ok"=w323:bool)  [unwired: 10 in]
              }
            }
            n101 = case shown="True" w316 {
              tunnel: w320 -> [w324 w333]
              tunnel: w319 -> [_ w332]
              tunnel: [w324 w326] -> w318
              frame False {
              }
              frame True {
                n102 = call "Sequence-Init.vi"("error in (no error)"=w333, "VariantSets"=w332) -> ("error out"=w331:errorcluster)  [unwired: 9 in]
                n103 = call "Station.Home.Check.vi"("error in (no error)"=w331) -> ("error out"=w327:errorcluster, "Homed?"=w330:bool)  [unwired: 6 in, 3 out]
                n104 = Select(t=Sequence.MainMode."Process" ("f"), s=w330, f=Sequence.MainMode."Base") -> (s? t:f=w325:T10)
                n105 = call "MainGui-ModeSelect.vi"("error in (no error)"=w327, "Mode"=w325) -> ("error out"=w326:errorcluster)  [unwired: 9 in]
              }
            }
          }
        }
      }
      frame "Init" {
        # "Station initialized after startup/EMG/Error/Stop. Station is not based (homing is needed to continue)"
        n106 = call "Station.Home.Check.vi"("error in (no error)"=w335) -> ("error out"=w338:errorcluster, "Error?"=w336:bool)  [unwired: 6 in, 3 out]
        n107 = call "FestoCPX.Station.ButtonsLed.Set.vi"("error in"=w338, "Buttons.State (OFF)"=T23 {"Start"=FALSE, "Stop"=FALSE, "Control"=TRUE} ("Buttons.State")) -> ("error out"=w341:errorcluster)  [unwired: 9 in]
        n108 = call "FestoCPX.Station.TowerLed.Set.vi"("error in"=w341, "Color (off)"=FestoCPX.Station.TowerLed.Color."off") -> ("error out"=w334:errorcluster)  [unwired: 9 in]
        n109 = Bundle By Name(cluster=w337, "State"=Station.State."Idle", "Hw failure"=w336) -> (w339:T2)
      }
      frame "Ready" {
        # "Station based (homed) - check for DUT only"
        n110 = call "FestoCPX.Station.ButtonsLed.Set.vi"("error in"=w345, "Buttons.State (OFF)"=T23 {"Start"=TRUE, "Stop"=FALSE, "Control"=TRUE} ("Buttons.State")) -> ("error out"=w346:errorcluster)  [unwired: 9 in]
        n111 = call "FestoCPX.Station.TowerLed.Set.vi"("error in"=w346, "Color (off)"=FestoCPX.Station.TowerLed.Color."green") -> ("error out"=w344:errorcluster)  [unwired: 9 in]
        n112 = Bundle By Name(cluster=w350, "State"=Station.State."Ready", "Home err"=FALSE) -> (w352:T2)
      }
      frame "Start" {
        # "Operator requests to start the sequence"
        n113 = global read "Config.Global.vi" "UserSets"() -> (w361:T9)
        n114 = Unbundle By Name(w361) -> ("Test.IgnoreResults"=w359:bool, "Test.IgnoreImages"=w363:bool, "Test.ServiceMode"=w358:bool)
        n115 = Compound Arithmetic op=OR(w359, w363, w358) -> (w355:bool)
        n116 = case shown="True" w355 {
          tunnel: [TRUE ("ok") w368] -> w357
          tunnel: Translator.Message."Test options are not set as default. Do you want to continue?" ("_Msg") -> [_ w367]
          frame False {
          }
          frame True {
            n117 = call "InfoGui.vi"("_Msg"=w367) -> ("ok"=w368:bool)  [unwired: 10 in]
          }
        }
        n118 = case shown="True" w357 {
          selector: w357 -> [w369 _]
          tunnel: [w369 w371] -> w356
          tunnel: [_ w370] -> w354
          frame False {
          }
          frame True {
            n119 = call "ProcessStartGui.vi"() -> ("ok"=w371:bool, "repeat?"=w370:bool)  [unwired: 10 in]
          }
        }
        n120 = case shown="True" w356 {
          tunnel: w365 -> [w373 w376]
          tunnel: [w373 w375] -> w364
          tunnel: w362 -> [w372 w379]
          tunnel: w361 -> [_ w378]
          tunnel: [w372 w377] -> w360
          tunnel: w354 -> [_ w374]
          frame False {
          }
          frame True {
            n121 = Bundle By Name(cluster=w379, "Sets"=w378, "Sets.ContinueOrder"=w374) -> (w377:T2)
            n122 = call "Station-Run.vi"("error in (no error)"=w376) -> ("error out"=w375:errorcluster)  [unwired: 10 in]
          }
        }
      }
      frame "Run" {
        n123 = Unbundle By Name(w387) -> ("Sets"=w386:T9)
        n124 = call "Sequence-Start.vi"("error in (no error)"=w388, "SeqOptions"=w386) -> ("error out"=w382:errorcluster)  [unwired: 9 in]
        n125 = global write "Station.Global.vi" "ProcStop"(FALSE ("ProcStop")) -> ()
        n126 = call "FestoCPX.Station.ButtonsLed.Set.vi"("error in"=w382, "Buttons.State (OFF)"=T23 {"Start"=FALSE, "Stop"=TRUE, "Control"=TRUE} ("Buttons.State")) -> ("error out"=w381:errorcluster)  [unwired: 9 in]
        n127 = Bundle By Name(cluster=w387, "State"=Station.State."Run") -> (w390:T2)
        n128 = call "FestoCPX.Station.TowerLed.Set.vi"("error in"=w381, "Color (off)"=FestoCPX.Station.TowerLed.Color."orange") -> ("error out"=w384:errorcluster)  [unwired: 9 in]
      }
      frame "Done" {
        n129 = call "FestoCPX.Station.ButtonsLed.Set.vi"("error in"=w399, "Buttons.State (OFF)"=T23 {"Start"=FALSE, "Stop"=FALSE, "Control"=TRUE} ("Buttons.State")) -> ("error out"=w393:errorcluster)  [unwired: 9 in]
        n130 = call "FestoCPX.Station.TowerHorn.Set.vi"("error in"=w393, "Horn (F)"=TRUE ("Horn1 (F)"), "Period [s] (0)"=3.0 ("Period [s]")) -> ("error out"=w392:errorcluster)  [unwired: 8 in]
        n131 = call "FestoCPX.Station.TowerLed.Set.vi"("error in"=w392, "Color (off)"=FestoCPX.Station.TowerLed.Color."green") -> ("error out"=w391:errorcluster)  [unwired: 9 in]
        n132 = Bundle By Name(cluster=w398, "State"=Station.State."Done") -> (w400:T2)
      }
      frame "Stop" {
        w406 = u32 500  # blink[ms]
        # "Operator requests to stop the sequence, set StopButtonOccurance to allow loops in step vis to stop"
        n133 = call "FestoCPX.Station.ButtonLed.On.vi"("error in"=w405, "Button Led"=FestoCPX.Station.ButtonLed."Stop", "Blink period [ms] (0)"=w406) -> ("error out"=w407:errorcluster)  [unwired: 8 in]
        n134 = call "Sequence-UserAction.vi"("error in (no error)"=w407, "UserAction"=Sequence.UserAction."Stop") -> ("error out"=w403:errorcluster)  [unwired: 9 in]
        n135 = Bundle By Name(cluster=w404, "State"=Station.State."Stop") -> (w410:T2)
      }
      frame "Error" {
        # "Sequence error occured"
        n136 = call "FestoCPX.Station.ButtonLed.Off.vi"("error in"=w417, "Button Led"=FestoCPX.Station.ButtonLed."Stop") -> ("error out"=w416:errorcluster)  [unwired: 9 in]
        n137 = call "FestoCPX.Station.TowerLed.Set.vi"("error in"=w416, "Color (off)"=FestoCPX.Station.TowerLed.Color."red", "Blink period [ms] (0)"=u32 500) -> ("error out"=w414:errorcluster)  [unwired: 8 in]
        n138 = call "FestoCPX.Station.TowerHorn.Set.vi"("error in"=w414, "Horn (F)"=TRUE ("Horn1 (F)"), "Period [s] (0)"=3.0 ("Period [s]")) -> ("error out"=w419:errorcluster)  [unwired: 8 in]
        n139 = Bundle By Name(cluster=w420, "State"=Station.State."Error", "Unconfirmed"=TRUE) -> (w421:T2)
      }
      frame "Home" {
        # "Start homing (basing)"
        n140 = call "Sequence-Home.vi"("error in (no error)"=w430) -> ("error out"=w425:errorcluster)  [unwired: 10 in]
        n141 = call "FestoCPX.Station.ButtonsLed.Set.vi"("error in"=w425, "Buttons.State (OFF)"=T23 {"Start"=FALSE, "Stop"=FALSE, "Control"=TRUE} ("Buttons.State")) -> ("error out"=w426:errorcluster)  [unwired: 9 in]
        n142 = call "FestoCPX.Station.TowerLed.Set.vi"("error in"=w426, "Color (off)"=FestoCPX.Station.TowerLed.Color."orange") -> ("error out"=w424:errorcluster)  [unwired: 9 in]
        n143 = Bundle By Name(cluster=w431, "State"=Station.State."Home", "Home err"=FALSE) -> (w433:T2)
      }
      frame "Seq.Run" {
        # "Sequence loop starts a process (work/step/home)"
        n144 = Unflatten From String(type=T26 {"State"=enum."Init", "PauseReason"=enum."-", "BreakSource"=enum."-"} ("cluster"), binary string=w443, error in (no error)=w444) -> (value=w440:T26, error out=w437:errorcluster)  [unwired: 2 in, 1 out]
        n145 = Unbundle By Name(w440) -> ("State"=w438:T4, "PauseReason"=w439:T5, "BreakSource"=w434:T6)
        n146 = Bundle By Name(cluster=w441, "Seq.State"=w438, "Seq.BreakReason"=w439, "Seq.BreakSource"=w434) -> (w442:T2)
        n147 = case shown="\"Pause\"" w438 {
          tunnel: w437 -> [w445 w447 w450]
          tunnel: [w445 w446 w454] -> w436
          frame Default {
          }
          frame "Run" {
            n148 = call "FestoCPX.Station.TowerLed.Set.vi"("error in"=w447, "Color (off)"=FestoCPX.Station.TowerLed.Color."orange") -> ("error out"=w446:errorcluster)  [unwired: 9 in]
          }
          frame "Pause" {
            n149 = call "FestoCPX.Station.TowerHorn.Set.vi"("error in"=w450, "Horn (F)"=TRUE ("Horn1 (F)"), "Period [s] (0)"=3.0 ("Period [s]")) -> ("error out"=w449:errorcluster)  [unwired: 8 in]
            n150 = call "FestoCPX.Station.TowerLed.Set.vi"("error in"=w449, "Color (off)"=FestoCPX.Station.TowerLed.Color."orange", "Blink period [ms] (0)"=u32 500) -> ("error out"=w454:errorcluster)  [unwired: 8 in]
          }
        }
      }
      frame "Seq.Done" {
        # "Sequence loop ends a process (work/step/home)"
        n151 = Unflatten From String(type=T28 {"State"=enum."Init", "Status"=enum."-", "order done"=FALSE} ("output cluster"), binary string=w466, error in (no error)=w467) -> (value=w464:T28, error out=w465:errorcluster)  [unwired: 2 in, 1 out]
        n152 = Unbundle By Name(w464) -> ("Status"=w462:T27, "State"=w460:T4, "order done"=w456:bool)
        n153 = case shown="\"Run\"" w460 {
          tunnel: w465 -> [w471 w484 w491]
          tunnel: [w470 w483 w491] -> w463
          tunnel: w462 -> [w469 w482 _]
          tunnel: [_ w481 _] -> w458
          tunnel: w456 -> [w468 _ _]
          frame "Run" {
            # "Test procedure done"
            n154 = case shown="Default" w469 {
              tunnel: w471 -> [w475 w480]
              tunnel: [w472 w479] -> w470
              tunnel: w468 -> [w474 _]
              frame Default {
                n155 = call "Station-Home.vi"("error in (no error)"=w475) -> ("error out"=w473:errorcluster)  [unwired: 10 in]
                n156 = case shown="False" w474 {
                  tunnel: w473 -> [w476 w478]
                  tunnel: [w476 w477] -> w472
                  frame False {
                  }
                  frame True {
                    n157 = call "ChangeOverGui-RefReject.vi"("error in"=w478) -> ("error out"=w477:errorcluster)  [unwired: 10 in]
                  }
                }
              }
              frame "Error", "Aborted" {
                # "Tester error"
                n158 = call "Station-Error.vi"("error in (no error)"=w480) -> ("error out"=w479:errorcluster)  [unwired: 10 in]
              }
            }
          }
          frame "Home" {
            # "Home procedure done"
            n159 = case shown="Default" w482 {
              tunnel: w484 -> [w486 w490]
              tunnel: [w487 w489] -> w483
              tunnel: [_ TRUE] -> w481
              frame Default {
                n160 = call "BaseGui-Done.vi"("error in"=w486) -> ("error out"=w485:errorcluster)  [unwired: 10 in]
                n161 = call "Station-Done.vi"("error in (no error)"=w485) -> ("error out"=w487:errorcluster)  [unwired: 10 in]
              }
              frame "Error", "Aborted" {
                # "Tester error"
                n162 = call "Station-Error.vi"("error in (no error)"=w490) -> ("error out"=w489:errorcluster)  [unwired: 10 in]
              }
            }
          }
          frame Default {
          }
        }
        n163 = Bundle By Name(cluster=w457, "Home err"=w458, "Seq.State"=w460) -> (w461:T2)
      }
      frame "Tower.Update" {
        # "Update tower (lights/horn/button lights)"
        n164 = call "FestoCPX.Station.TowerHorn.Fglb.vi"("Action (get)"=FestoCPX.Station.TowerHorn.Fglb.Action."get", "error in"=w502) -> ("error out"=w503:errorcluster, "Done?"=w504:bool)  [unwired: 8 in]
        n165 = case shown="True" w504 {
          tunnel: w503 -> [w514 w516]
          tunnel: [w514 w515] -> w501
          frame False {
          }
          frame True {
            # "Switch off the horn"
            n166 = call "FestoCPX.Station.TowerHorn.Set.vi"("error in"=w516) -> ("error out"=w515:errorcluster)  [unwired: 10 in]
          }
        }
        n167 = call "FestoCPX.Station.TowerLed.Fglb.vi"("error in"=w501) -> ("error out"=w499:errorcluster, "Trigger"=w500:bool, "Color out"=w498:T13)  [unwired: 8 in]
        n168 = case shown="False" w500 {
          tunnel: w499 -> [w510 w513]
          tunnel: [w510 w512] -> w495
          tunnel: w498 -> [_ w511]
          frame False {
          }
          frame True {
            # "Blink the tower light"
            n169 = call "FestoCPX.Station.TowerLed.Update.vi"("error in"=w513, "Color (off)"=w511) -> ("error out"=w512:errorcluster)  [unwired: 9 in]
          }
        }
        n170 = call "FestoCPX.Station.ButtonLed.Fglb.vi"("error in"=w495) -> ("error out"=w497:errorcluster, "Trigger"=w496:bool, "State"=w493:T23)  [unwired: 8 in]
        n171 = case shown="True" w496 {
          tunnel: w497 -> [w506 w509]
          tunnel: [w506 w508] -> w494
          tunnel: w493 -> [_ w507]
          frame False {
          }
          frame True {
            # "Blink the button's light"
            n172 = call "FestoCPX.Station.ButtonsLed.Update.vi"("error in"=w509, "Buttons.State"=w507) -> ("error out"=w508:errorcluster)  [unwired: 9 in]
          }
        }
      }
      frame "Mode.Select" {
        # "Operator selects the mode (Auto/Step/CG)"
        n173 = Unflatten From String(type=T9 {"GuiMode"=enum."Process", "Test"={"IgnoreResults"=FALSE, "IgnoreImages"=FALSE, "ServiceMode"=FALSE}, "ContinueOrder"=FALSE} ("SeqOptions"), binary string=w525, error in (no error)=w526) -> (value=w522:T9, error out=w524:errorcluster)  [unwired: 2 in, 1 out]
        n174 = Unbundle By Name(w522) -> ("GuiMode"=w521:T10)
        n175 = call "Sequence-UserData.vi"("error in (no error)"=w524, "SeqOptions"=w522) -> ("error out"=w519:errorcluster)  [unwired: 9 in]
        n176 = Bundle By Name(cluster=w523, "Sets"=w522) -> (w518:T2)
        n177 = Unbundle By Name(w518) -> ("State"=w517:T3)
        n178 = disable-structure shown="Enabled" {
          disable-tunnel: w521 -> [w531 _]
          disable-tunnel: [w530 w542] -> w520
          disable-tunnel: w519 -> [w529 w542]
          disable-tunnel: w517 -> [w528 _]
          frame Disabled {
            n179 = case shown="\"Idle\", \"Ready\"" w528 {
              tunnel: w531 -> [_ w535]
              tunnel: [w532 w534] -> w530
              tunnel: w529 -> [w532 w533]
              frame Default {
              }
              frame "Idle", "Ready" {
                n180 = case shown="Default" w535 {
                  tunnel: w533 -> [w538 w541]
                  tunnel: [w537 w539] -> w534
                  frame Default {
                    n181 = call "FestoCPX.Station.TowerLed.Set.vi"("error in"=w538, "Color (off)"=FestoCPX.Station.TowerLed.Color."green") -> ("error out"=w537:errorcluster)  [unwired: 9 in]
                  }
                  frame "Order" {
                    n182 = call "FestoCPX.Station.TowerLed.Set.vi"("error in"=w541, "Color (off)"=FestoCPX.Station.TowerLed.Color."green/orange") -> ("error out"=w539:errorcluster)  [unwired: 9 in]
                  }
                }
              }
            }
          }
          frame Enabled {
          }
        }
      }
      frame "Emg" {
        # "Emergency circuit occurance (Emg Button/Safety Bar) - ask to press control button to restart the emergency circuit"
        n183 = Unbundle By Name(w548) -> ("State"=w552:T3, "EmgState"=w543:T8)
        n184 = Cluster To Array(cluster=w543) -> (array=w544:bool[])
        n185 = Or Array Elements(Boolean array=w544) -> (logical OR=w550:bool)
        n186 = case shown="True" w550 {
          tunnel: [w555 w561] -> w551
          tunnel: w549 -> [w555 w558]
          frame False {
          }
          frame True {
            n187 = call "FestoCPX.Station.TowerLed.Set.vi"("error in"=w558, "Color (off)"=FestoCPX.Station.TowerLed.Color."red", "Blink period [ms] (0)"=u32 500) -> ("error out"=w557:errorcluster)  [unwired: 8 in]
            n188 = call "FestoCPX.Station.ButtonLed.Off.vi"("error in"=w557, "Button Led"=FestoCPX.Station.ButtonLed."Control") -> ("error out"=w561:errorcluster)  [unwired: 9 in]
          }
        }
        n189 = call "FestoCPX.Station.TowerHorn.Set.vi"("Horn (F)"=TRUE ("Horn1 (F)"), "Period [s] (0)"=3.0 ("Period [s]")) -> ()  [unwired: 9 in, 1 out]
        n190 = case shown="\"Run\", \"Home\"" w552 {
          tunnel: w551 -> [w562 w564]
          tunnel: [w562 w563] -> w547
          frame Default {
          }
          frame "Run", "Home" {
            n191 = call "Sequence-Abort.vi"("error in (no error)"=w564) -> ("error out"=w563:errorcluster)  [unwired: 10 in]
          }
        }
        n192 = Bundle By Name(cluster=w548, "State"=Station.State."Emg") -> (w554:T2)
      }
      frame "Emg.Reset" {
        # "Try to reset emergency circuit - if ok then initialize the station"
        n193 = call "FestoCPX.Station.Emg.Reset.vi"("error in"=w568) -> ("error out"=w567:errorcluster)  [unwired: 10 in]
        n194 = call "Station-Home.vi"("error in (no error)"=w567) -> ("error out"=w565:errorcluster)  [unwired: 10 in]
        n195 = case shown="No Error" w565 {
          selector: w565 -> [w572 w577]
          tunnel: w570 -> [w576 w578]
          tunnel: [w575 w578] -> w569
          tunnel: [w571 w577] -> w566
          frame No Error {
            n196 = Bundle By Name(cluster=w576, "EmgState"=T8 {"Button"=FALSE, "SideDoor"=FALSE, "FrontDoor"=FALSE, "DoorSecured"=FALSE}) -> (w575:T2)
            n197 = call "FestoCPX.Station.Door.Lock.vi"("error in"=w572, "Lock"=FALSE) -> ("error out"=w571:errorcluster)  [unwired: 9 in]
          }
          frame Error {
          }
        }
      }
      frame "Emg.Check" {
        # "Check for emergency circuit state"
        n198 = Unbundle By Name(w583) -> ("State"=w584:T3, "Seq.State"=w580:T4)
        n199 = call "FestoCPX.Station.Emg.Check.vi"("error in"=w587) -> ("error out"=w586:errorcluster, "Emg"=w581:T8)  [unwired: 8 in, 1 out]
        n200 = case shown="Default" w580 {
          tunnel: w581 -> [w591 w596]
          tunnel: [w588 w593] -> w579
          frame Default {
            n201 = Unbundle(w591) -> ("Button"=w590:bool, "SideDoor"=w589:bool)  [unwired: 2 out]
            n202 = Compound Arithmetic op=OR(w590, w589) -> (w588:bool)
          }
          frame "Run" {
            n203 = Unbundle(w596) -> ("Button"=w595:bool, "SideDoor"=w594:bool, "FrontDoor"=w592:bool)  [unwired: 1 out]
            n204 = Compound Arithmetic op=OR(w595, w594, w592) -> (w593:bool)
          }
        }
        n205 = case shown="Default" w584 {
          tunnel: w586 -> [w597 w600]
          tunnel: [w597 w599] -> w585
          tunnel: w579 -> [_ w598]
          frame "Emg" {
          }
          frame Default {
            n206 = case shown="True" w598 {
              tunnel: w600 -> [w601 w603]
              tunnel: [w601 w602] -> w599
              frame False {
              }
              frame True {
                # "Emergency button pressed or door open"
                n207 = call "Station-Emg.vi"("error in (no error)"=w603) -> ("error out"=w602:errorcluster)  [unwired: 10 in]
              }
            }
          }
        }
        n208 = Bundle By Name(cluster=w583, "EmgState"=w581) -> (w582:T2)
      }
      frame "Home.Check" {
        n209 = global read "Station.Global.vi" "Changeover state"() -> (w604:T19)
        n210 = Unbundle By Name(w612) -> ("State"=w608:T3)
        n211 = call "Station.Home.Check.vi"("error in (no error)"=w613) -> ("error out"=w606:errorcluster, "Homed?"=w607:bool, "Error?"=w609:bool, "Station Home Status"=w605:T12)  [unwired: 6 in, 1 out]
        n212 = case shown="\"Done\"" w608 {
          tunnel: w606 -> [w615 w627 w632 w638]
          tunnel: [w617 w628 w634 w638] -> w610
          tunnel: w607 -> [w616 _ w633 _]
          tunnel: w605 -> [_ w626 _ _]
          tunnel: w604 -> [w614 _ _ _]
          frame "Idle" {
            n213 = case shown="\"Ready\"" w614 {
              tunnel: [w618 w621] -> w617
              tunnel: w616 -> [_ w620]
              tunnel: w615 -> [w618 w619]
              frame Default {
              }
              frame "Ready" {
                n214 = case shown="True" w620 {
                  tunnel: w619 -> [w622 w624]
                  tunnel: [w622 w623] -> w621
                  frame False {
                  }
                  frame True {
                    n215 = call "Station-Ready.vi"("error in (no error)"=w624) -> ("error out"=w623:errorcluster)  [unwired: 10 in]
                  }
                }
              }
            }
          }
          frame "Done" {
            n216 = Unbundle By Name(w626) -> ()  [unwired: 1 out]
            n217 = case shown="False" FALSE {
              tunnel: w627 -> [w630 w631]
              tunnel: [w629 w631] -> w628
              frame False {
                n218 = call "Station-Init.vi"("error in (no error)"=w630) -> ("error out"=w629:errorcluster)  [unwired: 10 in]
              }
              frame True {
              }
            }
          }
          frame "Ready" {
            n219 = case shown="False" w633 {
              tunnel: w632 -> [w636 w637]
              tunnel: [w635 w637] -> w634
              frame False {
                n220 = call "Station-Init.vi"("error in (no error)"=w636) -> ("error out"=w635:errorcluster)  [unwired: 10 in]
              }
              frame True {
              }
            }
          }
          frame Default {
          }
        }
        n221 = Bundle By Name(cluster=w612, "StatusBits"=w605, "Hw failure"=w609) -> (w611:T2)
      }
      frame "Prod.Check" {
        # "Check DUT's presence in the tester and barcode scanning status"
        n222 = call "FestoCPX.Station.ProdPresent.Check.vi"("error in"=w643) -> ("error out"=w642:errorcluster, "Prod Present"=w639:T7)  [unwired: 5 in, 4 out]
        n223 = Bundle By Name(cluster=w640, "DUT present"=w639) -> (w641:T2)
      }
      frame "Butt.Check" {
        w647 = T19[] [enum."Init", enum."Ready"] items=["Init", "Scaning", "NOK", "Wait for ack", "Ready"]
        # "Check the hardware buttons"
        n224 = call "Station.Buttons.Check.vi"("error in"=w663) -> ("error out"=w660:errorcluster, "Buttons array"=w650:bool[], "Buttons"=w651:T41)  [unwired: 8 in]
        n225 = Unbundle By Name(w649) -> ("Hw failure"=w652:bool, "Unconfirmed"=w655:bool, "State"=w662:T3, "Sets.GuiMode"=w654:T10, "StatusBits.Door Close"=w648:bool)
        n226 = global read "Station.Global.vi" "Changeover state"() -> (w644:T19)
        n227 = feedback-in #2(w651) -> ()
        n228 = feedback #2(w651) -> (w657:T41)
        n229 = Or Array Elements(Boolean array=w650) -> ()  [unwired: 1 out]
        n230 = Compound Arithmetic op=AND(invert w657, w651) -> (w656:T41)
        n231 = Unbundle By Name(w656) -> ("Start"=w661:bool, "Stop"=w659:bool, "Control"=w658:bool)
        n232 = Equal?(x=w644, y=w647) -> (x = y?=w646:bool[])
        n233 = Or Array Elements(Boolean array=w646) -> (logical OR=w645:bool)
        n234 = case shown="\"Run\"" w662 {
          tunnel: w661 -> [w668 w692 w714 _ _]
          tunnel: w660 -> [w671 w695 w715 w725 w729]
          tunnel: w659 -> [_ _ w711 _ _]
          tunnel: w658 -> [_ _ _ w723 _]
          tunnel: w655 -> [w666 _ _ _ _]
          tunnel: w654 -> [w669 w693 w713 _ _]
          tunnel: [w670 w694 w712 w724 w729] -> w653
          tunnel: w652 -> [w665 _ _ _ _]
          tunnel: w648 -> [w667 _ _ _ _]
          tunnel: w645 -> [w664 w691 _ _ _]
          frame "Idle" {
            n235 = case shown="\"Order\"" w669 {
              tunnel: w671 -> [w672 w679 w687]
              tunnel: [w672 w678 w686] -> w670
              tunnel: w668 -> [_ w677 w683]
              tunnel: w667 -> [_ w676 _]
              tunnel: w666 -> [_ w675 _]
              tunnel: w665 -> [_ w674 _]
              tunnel: w664 -> [_ _ w684]
              frame Default {
              }
              frame "Base" {
                n236 = Compound Arithmetic op=AND(invert w674, invert w675, w676, w677) -> (w673:bool)
                n237 = case shown="True" w673 {
                  tunnel: w679 -> [w680 w682]
                  tunnel: [w680 w681] -> w678
                  frame False {
                  }
                  frame True {
                    # "Start Base procedure"
                    n238 = call "Station-Home.vi"("error in (no error)"=w682) -> ("error out"=w681:errorcluster)  [unwired: 10 in]
                  }
                }
              }
              frame "Order" {
                n239 = Compound Arithmetic op=AND(w684, w683) -> (w685:bool)
                n240 = case shown="True" w685 {
                  tunnel: w687 -> [w688 w690]
                  tunnel: [w688 w689] -> w686
                  frame False {
                  }
                  frame True {
                    # "Scan new order"
                    n241 = call "ChangeOverGui-Scan.vi"("error in"=w690) -> ("error out"=w689:errorcluster)  [unwired: 10 in]
                  }
                }
              }
            }
          }
          frame "Ready" {
            n242 = case shown="\"Process\", \"Base\"" w693 {
              tunnel: w692 -> [_ w697 w705]
              tunnel: w695 -> [w696 w700 w707]
              tunnel: [w696 w699 w706] -> w694
              tunnel: w691 -> [_ w698 _]
              frame Default {
              }
              frame "Order" {
                n243 = Compound Arithmetic op=AND(w698, w697) -> (w701:bool)
                n244 = case shown="True" w701 {
                  tunnel: w700 -> [w702 w704]
                  tunnel: [w702 w703] -> w699
                  frame False {
                  }
                  frame True {
                    # "Scan new order"
                    n245 = call "ChangeOverGui-Scan.vi"("error in"=w704) -> ("error out"=w703:errorcluster)  [unwired: 10 in]
                  }
                }
              }
              frame "Process", "Base" {
                n246 = case shown="True" w705 {
                  tunnel: w707 -> [w708 w710]
                  tunnel: [w708 w709] -> w706
                  frame False {
                  }
                  frame True {
                    # "Start sequence"
                    n247 = call "Station-Start.vi"("error in (no error)"=w710) -> ("error out"=w709:errorcluster)  [unwired: 10 in]
                  }
                }
              }
            }
          }
          frame "Run" {
            n248 = case shown="\"Process\", \"Base\"" w713 {
              tunnel: w714 -> [_ _]
              tunnel: w715 -> [w716 w719]
              tunnel: [w716 w718] -> w712
              tunnel: w711 -> [_ w717]
              frame Default {
              }
              frame "Process", "Base" {
                n249 = case shown="False" w717 {
                  tunnel: w719 -> [w720 w722]
                  tunnel: [w720 w721] -> w718
                  frame False {
                  }
                  frame True {
                    # "Stop the sequence"
                    n250 = call "Station-Stop.vi"("error in (no error)"=w722) -> ("error out"=w721:errorcluster)  [unwired: 10 in]
                  }
                }
              }
            }
          }
          frame "Emg" {
            n251 = case shown="True" w723 {
              tunnel: w725 -> [w726 w728]
              tunnel: [w726 w727] -> w724
              frame False {
              }
              frame True {
                # "Reset EMG error"
                n252 = call "Station-EmgReset.vi"("error in (no error)"=w728) -> ("error out"=w727:errorcluster)  [unwired: 10 in]
              }
            }
          }
          frame Default {
          }
        }
      }
    }
    "Data" <- w2
    n253 = global write "Station.Global.vi" "Station"(w2) -> ()
    n254 = call "citTemplate.sendAckNotifier.vi"("notification data"=w11, "notifierHandle in"=w12, "error in"=w1) -> ()  [unwired: 13 out]
    n255 = call "citTemplate.ErrorEventPass.vi"("error in"=w1, "action of error"=w6, "event in"=w10) -> ("error out"=w5:errorcluster)  [unwired: 2 in, 6 out]
  }
  n256 = disable-structure shown="Disabled" {
    frame Disabled {
      (unwired) Station.State."Error" ("State")
      # "Put important VIs here..."
      n257 = call "citTemplate.clearQueue.vi"() -> ()  [unwired: 14 in, 2 out]
      n258 = call "citTemplate.writeQueue.vi"() -> ()  [unwired: 15 in, 1 out]
      n259 = call "citTemplate.writeQueueWithAck.vi"() -> ()  [unwired: 13 in, 3 out]
      n260 = call "citTemplate.ErrorEventPass.vi"() -> ()  [unwired: 11 in, 1 out]
      n261 = Flatten To String() -> ()  [unwired: 4 in, 3 out]
      n262 = Unflatten From String() -> ()  [unwired: 5 in, 3 out]
      n263 = call "FestoCPX.Station.ButtonLed.On.vi"() -> ()  [unwired: 11 in, 1 out]
      n264 = call "Station.Home.Check.vi"() -> ()  [unwired: 7 in, 5 out]
      n265 = call "FestoCPX.Station.ButtonLed.Off.vi"() -> ()  [unwired: 11 in, 1 out]
      n266 = call "FestoCPX.Station.TowerHorn.Set.vi"() -> ()  [unwired: 11 in, 1 out]
      n267 = call "FestoCPX.Station.ButtonsLed.Set.vi"() -> ()  [unwired: 11 in, 1 out]
      n268 = call "FestoCPX.Station.TowerLed.Set.vi"() -> ()  [unwired: 11 in, 1 out]
      n269 = call "Station-Error.vi"() -> ()  [unwired: 11 in, 1 out]
      n270 = call "Station-Init.vi"() -> ()  [unwired: 11 in, 1 out]
      n271 = call "Station-EmgCheck.vi"() -> ()  [unwired: 11 in, 1 out]
      n272 = call "Station-EmgReset.vi"() -> ()  [unwired: 11 in, 1 out]
      n273 = call "Station-ButtonsCheck.vi"() -> ()  [unwired: 11 in, 1 out]
      n274 = call "Station-Start.vi"() -> ()  [unwired: 11 in, 1 out]
      n275 = call "Station-Stop.vi"() -> ()  [unwired: 11 in, 1 out]
      n276 = call "Station-Emg.vi"() -> ()  [unwired: 11 in, 1 out]
      n277 = call "Station-ProdCheck.vi"() -> ()  [unwired: 11 in, 1 out]
      n278 = call "Station-Order.vi"() -> ()  [unwired: 11 in, 1 out]
      n279 = call "Station-Home.vi"() -> ()  [unwired: 11 in, 1 out]
      n280 = call "Station-SeqDone.vi"() -> ()  [unwired: 11 in, 1 out]
      n281 = call "Station-Done.vi"() -> ()  [unwired: 11 in, 1 out]
      n282 = call "Station-Ready.vi"() -> ()  [unwired: 11 in, 1 out]
      n283 = call "Station-StatusClear.vi"() -> ()  [unwired: 11 in, 1 out]
      n284 = call "Station-SeqRun.vi"() -> ()  [unwired: 11 in, 1 out]
      n285 = call "Station-StatusUpdate.vi"() -> ()  [unwired: 11 in, 1 out]
      n286 = call "Station-ModeSelect.vi"() -> ()  [unwired: 11 in, 1 out]
    }
    frame Enabled {
    }
  }
